vi "ZLIB Common Path to Specific Path.vi"(10 "common path":string) -> (2 "specific path":path)   [LabVIEW 2014]
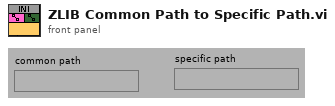
[diagram p1: front panel]
types:
  T1 = enum32{"invalid OS target", "Mac OS", "Windows 3.1", "Windows 95/NT", "Solaris 1", "Solaris 2", "HP-UX", "PowerMAX", "Linux", "Irix", "Rhapsody", "BeOS", "AIX", "OSF1", "VxWorks", "PharLap", "Carbon", "RTX", "Windows x64", "Linux x64", "Mac OS X x64"}
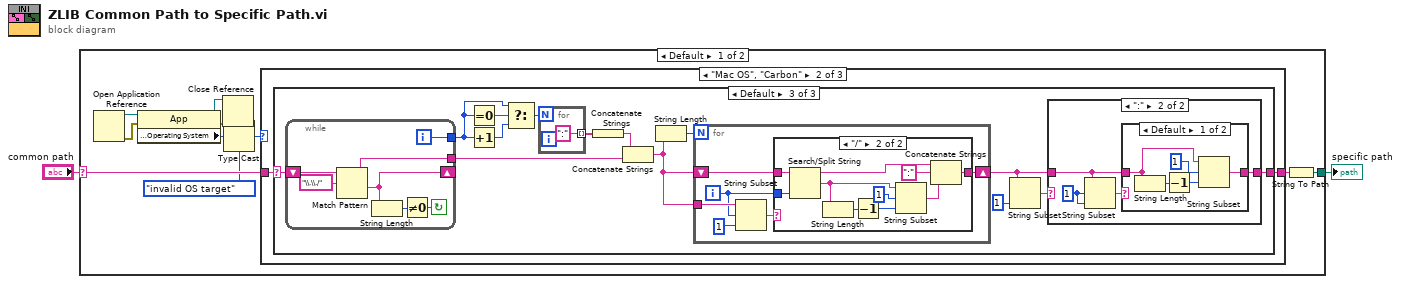
[diagram p0: block diagram]
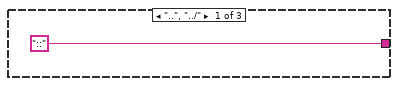
[diagram p3: hidden frame]
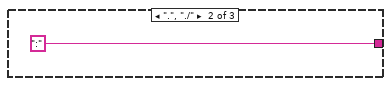
[diagram p4: hidden frame]
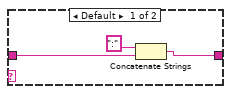
[diagram p6: hidden frame]
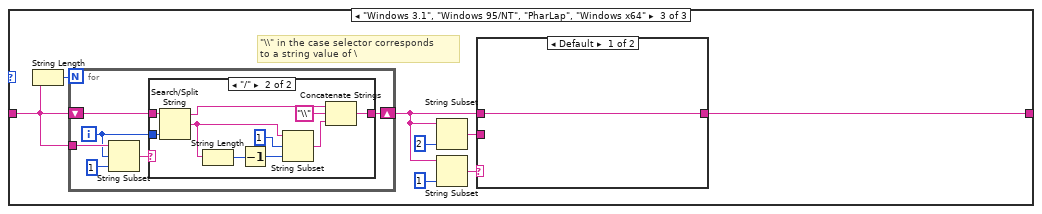
[diagram p8: hidden frame]
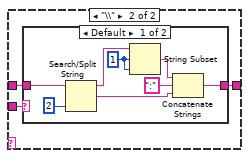
[diagram p10: hidden frame]
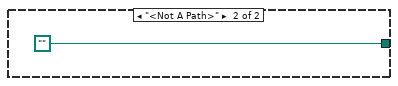
[diagram p12: hidden frame]
diagram:
  n1 = case shown="Default" "common path" {
    selector: "common path" -> [w12 _]
    tunnel: [w11 path "" ("Not A Path Constant")] -> w1
    frame Default {
      n2 = Open Application Reference() -> (0:w6:errorcluster, 3:w7:refnum<vi>)  [unwired: 4 in]
      n3 = property class="App"(reference=w7, error in=w6) -> (reference out=w8:refnum<vi>, error out=w9:errorcluster, "Application:Target:Operating System"=w4:T1)
      n4 = Close Reference(reference=w8, error in (no error)=w9) -> ()  [unwired: 1 out]
      n5 = Type Cast(type=T1."invalid OS target" ("Application:Target Operating System"), x=w4) -> (*(type *) &x=w3:T1)
      n6 = case shown="\"Mac OS\", \"Carbon\"" w3 {
        tunnel: w12 -> [w13 w15 w77]
        tunnel: [w13 w14 w75] -> w10
        frame "Linux", "VxWorks", "Linux x64", Default {
        }
        frame "Mac OS", "Carbon" {
          n7 = case shown="Default" w15 {
            selector: w15 -> [_ _ w21]
            tunnel: ["::" ":" w20] -> w14
            frame "..", "../" {
            }
            frame ".", "./" {
            }
            frame Default {
              n8 = while {
                shift-right: [w33] -> _
                shift-left: w21 -> [w37]
                tunnel: [w34] -> w25
                tunnel: [w32] -> w29
                i -> [w32]
                stop <- w35 continue-if-true
                n9 = Match Pattern(string=w37, regular expression="\\.\\./") -> (before substring=w34:string, after substring=w33:string)  [unwired: 3 out]
                n10 = String Length(string=w33) -> (length=w36:i32)
                n11 = Not Equal To 0?(x=w36) -> (x != 0?=w35:bool)
              }
              n12 = Equal To 0?(x=w29) -> (x = 0?=w30:bool)
              n13 = Increment(x=w29) -> (x+1=w28:i32)
              n14 = Select(t=w29, s=w30, f=w28) -> (s? t:f=w27:i32)
              n15 = for {
                N: w27 -> [_]
                tunnel: [":"] -> w26 mode=indexing
              }
              n16 = Concatenate Strings(w26) -> (w19:string)
              n17 = Concatenate Strings(w19, w25) -> (w23:string)
              n18 = String Length(string=w23) -> (length=w24:i32)
              n19 = for {
                N: w24 -> [_]
                tunnel: w23 -> [w42]
                shift-right: [w43] -> w18
                shift-left: w23 -> [w44]
                i -> [w41]
                n20 = String Subset(string=w42, offset (0)=w41, length (rest)=1 ("length")) -> (substring=w39:string)
                n21 = case shown="\"/\"" w39 {
                  tunnel: w44 -> [w45 w55]
                  tunnel: w41 -> [_ w48]
                  tunnel: [w45 w53] -> w43
                  frame Default {
                  }
                  frame "/" {
                    n22 = Search/Split String(string=w55, offset (0)=w48) -> (substring before match=w54:string, match + rest of string=w47:string)  [unwired: 2 out]
                    n23 = String Length(string=w47) -> (length=w51:i32)
                    n24 = Decrement(x=w51) -> (x-1=w50:i32)
                    n25 = String Subset(string=w47, offset (0)=1, length (rest)=w50) -> (substring=w46:string)
                    n26 = Concatenate Strings(w54, ":" ("x"), w46) -> (w53:string)
                  }
                }
              }
              n27 = String Subset(string=w18, length (rest)=1 ("length")) -> (substring=w22:string)  [unwired: 1 out]
              n28 = case shown="\":\"" w22 {
                tunnel: w18 -> [w59 w62]
                tunnel: [w58 w63] -> w20
                frame Default {
                  n29 = Concatenate Strings(":", w59) -> (w58:string)
                }
                frame ":" {
                  w61 = 1 ("length")
                  n30 = String Subset(string=w62, offset (0)=w61, length (rest)=w61) -> (substring=w60:string)
                  n31 = case shown="Default" w60 {
                    tunnel: w62 -> [w64 w69]
                    tunnel: [w65 w69] -> w63
                    frame Default {
                      n32 = String Length(string=w64) -> (length=w67:i32)
                      n33 = Decrement(x=w67) -> (x-1=w66:i32)
                      n34 = String Subset(string=w64, offset (0)=1, length (rest)=w66) -> (substring=w65:string)
                    }
                    frame ":" {
                    }
                  }
                }
              }
            }
          }
        }
        frame "Windows 3.1", "Windows 95/NT", "PharLap", "Windows x64" {
          # "\"\\\\\" in the case selector corresponds\nto a string value of \\"
          n35 = String Length(string=w77) -> (length=w73:i32)
          n36 = for {
            N: w73 -> [_]
            tunnel: w77 -> [w81]
            shift-right: [w82] -> w72
            shift-left: w77 -> [w83]
            i -> [w80]
            n37 = String Subset(string=w81, offset (0)=w80, length (rest)=1 ("length")) -> (substring=w78:string)
            n38 = case shown="\"/\"" w78 {
              tunnel: w83 -> [w84 w94]
              tunnel: w80 -> [_ w86]
              tunnel: [w84 w92] -> w82
              frame Default {
              }
              frame "/" {
                n39 = Search/Split String(string=w94, offset (0)=w86) -> (substring before match=w93:string, match + rest of string=w90:string)  [unwired: 2 out]
                n40 = String Length(string=w90) -> (length=w89:i32)
                n41 = Decrement(x=w89) -> (x-1=w88:i32)
                n42 = String Subset(string=w90, offset (0)=1, length (rest)=w88) -> (substring=w85:string)
                n43 = Concatenate Strings(w93, "\\" ("x"), w85) -> (w92:string)
              }
            }
          }
          n44 = String Subset(string=w72, length (rest)=2 ("length")) -> (substring=w70:string)  [unwired: 1 out]
          n45 = String Subset(string=w72, length (rest)=1 ("length")) -> (substring=w71:string)  [unwired: 1 out]
          n46 = case shown="Default" w71 {
            tunnel: w72 -> [w95 w98]
            tunnel: [w95 w97] -> w75
            tunnel: w70 -> [_ w96]
            frame Default {
            }
            frame "\\" {
              n47 = case shown="Default" w96 {
                tunnel: w98 -> [w106 w107]
                tunnel: [w100 w107] -> w97
                frame Default {
                  w99 = 1 ("offset (0)")
                  n48 = Search/Split String(string=w106, offset (0)=2) -> (substring before match=w104:string, match + rest of string=w101:string)  [unwired: 2 out]
                  n49 = String Subset(string=w104, offset (0)=w99, length (rest)=w99) -> (substring=w103:string)
                  n50 = Concatenate Strings(w103, ":", w101) -> (w100:string)
                }
                frame "\\\\" {
                  # "\"\\\\\\\\\" in the case selector corresponds\nto a string value of \\\\"
                }
              }
            }
          }
        }
      }
      n51 = String To Path(string=w10) -> (path=w11:path)
    }
    frame "<Not A Path>" {
    }
  }
  "specific path" <- w1
